vi "loadDaily.vi"(9 "end date":string, 11 "begin date":string) -> (0 "error out":errorcluster)   [LabVIEW 2012]
uses:
  <vilib>/addons/database/Auxilliary.llb/DB Tools Cursor Type.ctl
  Global1.vi
  <vilib>/addons/database/Connection.llb/DB Tools Open Connec (Path).vi
  <vilib>/addons/database/Connection.llb/Conn Execute.vi
  <vilib>/addons/database/Recordset.llb/Rec Destroy - Connection.vi
  <vilib>/addons/database/NI_Database_API.lvlib
panel:
  in  "error in (no error)":errorcluster
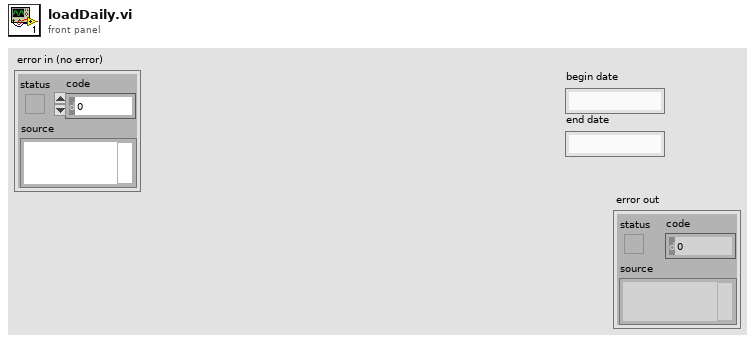
[diagram p1: front panel]
types:
  T1 = typedef "NI_Database_API.lvlib/DB Tools Cursor Type.ctl" = enum16{"forward-only", "keyset", "dynamic", "static"}
  T2 = typedef "NI_Database_API.lvlib/Conn ObjectReference.ctl" = refnum<k1>
  T3 = typedef "NI_Database_API.lvlib/Rec ObjectReference.ctl" = refnum<k1>
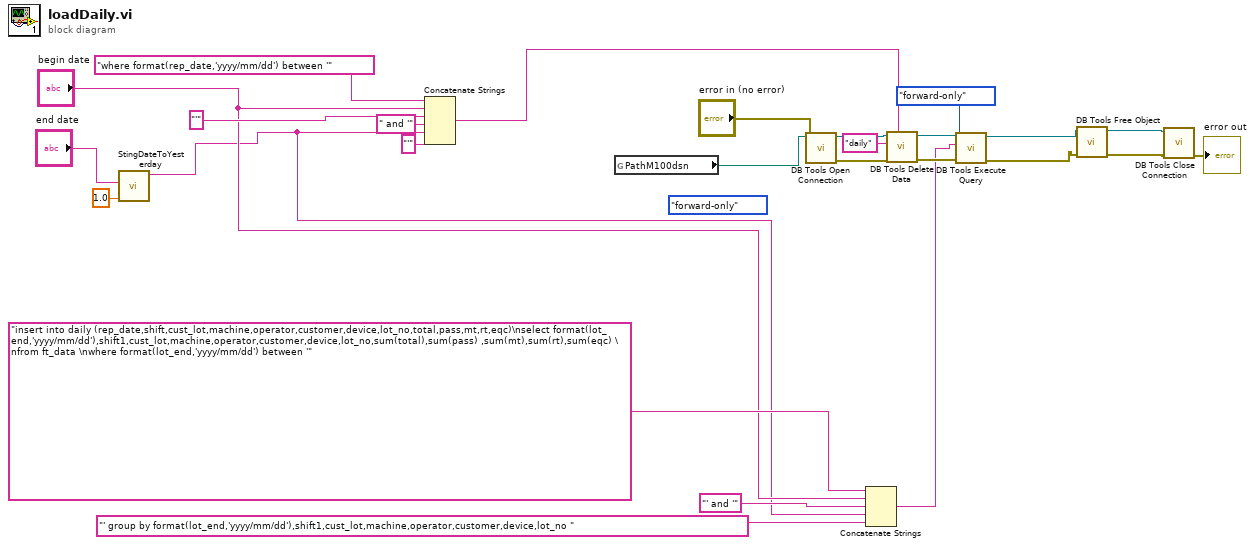
[diagram p0: block diagram]
diagram:
  (unwired) DB_Tools_Cursor_Type."forward-only" ("cursor type")
  n1 = call "StingDateToYesterday.vi"("Days"=1.0, "Date"="end date") -> ("Date+1"=w1:string)  [unwired: 8 in, 1 out]
  n2 = Concatenate Strings("where format(rep_date,'yyyy/mm/dd') between '" ("string"), "begin date", "'" ("string"), " and '" ("string"), w1, "'" ("string")) -> (w18:string)
  n3 = global read "Global1.vi" "PathM100dsn"() -> (w4:path)
  n4 = call-poly <vilib>:"DB Tools Open Connection.vi"("error in (no error)"="error in (no error)", "connection information"=w4) -> ("error out"=w23:errorcluster, "connection reference"=w24:T2)  [unwired: 6 in]
  n5 = Concatenate Strings("insert into daily (rep_date,shift,cust_lot,machine,operator,customer,device,lot_no,total,pass,mt,rt,eqc)\nselect format(lot_end,'yyyy/mm/dd'),shift1,cust_lot,machine,operator,customer,device,lot_no,sum(total),sum(pass) ,sum(mt),sum(rt),sum(eqc) \nfrom ft_data \nwhere format(lot_end,'yyyy/mm/dd') between '" ("string"), "begin date", "' and '" ("string"), w1, "' group by format(lot_end,'yyyy/mm/dd'),shift1,cust_lot,machine,operator,customer,device,lot_no " ("string")) -> (w6:string)
  n6 = call <vilib>:"DB Tools Delete Data.vi"("condition"=w18, "error in (no error)"=w23, "table"="daily", "connection reference"=w24) -> ("error out"=w7:errorcluster, "connection reference out"=w8:T2)  [unwired: 6 in]
  n7 = call-poly <vilib>:"DB Tools Execute Query.vi"("error in (no error)"=w7, "cursor type"=DB_Tools_Cursor_Type."forward-only", "SQL query"=w6, "connection reference"=w8) -> ("error out"=w9:errorcluster, "recordset reference"=w10:T3)  [unwired: 4 in]
  n8 = call-poly <vilib>:"DB Tools Free Object.vi"("error in (no error)"=w9, "recordset reference"=w10) -> ("error out"=w11:errorcluster, "connection reference"=w12:T2)  [unwired: 8 in]
  n9 = call <vilib>:"DB Tools Close Connection.vi"("error in (no error)"=w11, "connection reference"=w12) -> ("error out"=→"error out":errorcluster)  [unwired: 5 in]
